vi "Build Path to Macro.vi"(9 "Macro Name":string, 11 "App Data Dir":path) -> (2 "Macro File Path":path)   [LabVIEW 2023]
doc: "Builds the path to a macro file using the provided inputs."
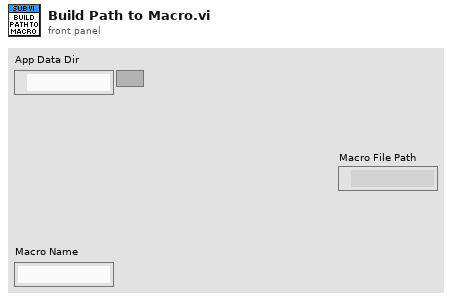
[diagram p1: front panel]
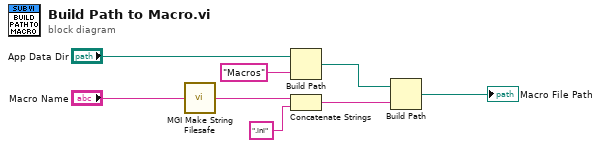
[diagram p0: block diagram]
diagram:
  n1 = call <userlib>:"MGI Make String Filesafe.vi"("String In"="Macro Name") -> ("Filesafe String Out"=w1:string)
  n2 = Build Path(base path="App Data Dir", name or relative path="Macros" ("string")) -> (appended path=w5:path)
  n3 = Concatenate Strings(w1, ".ini" ("string")) -> (w7:string)
  n4 = Build Path(base path=w5, name or relative path=w7) -> (appended path=→"Macro File Path":path)
